vi "ForceGraph(Position).vi"(8 "number":dbl, 9 "Setpoint":dbl, 10 "k":dbl, 11 "Function":string) -> (1 "force":dbl)   [LabVIEW 2023]
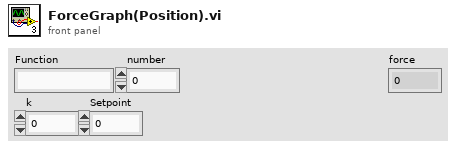
[diagram p1: front panel]
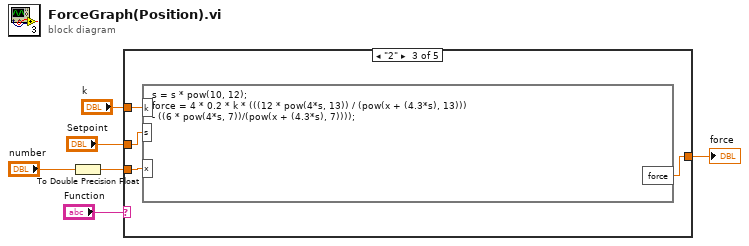
[diagram p0: block diagram]
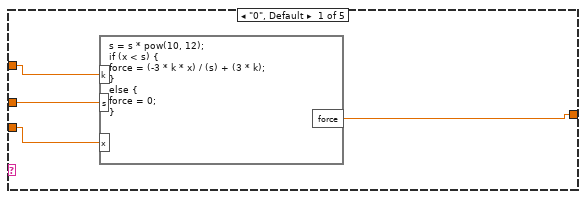
[diagram p2: hidden frame]
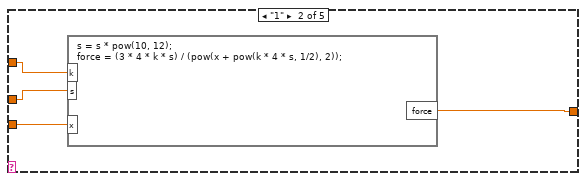
[diagram p3: hidden frame]
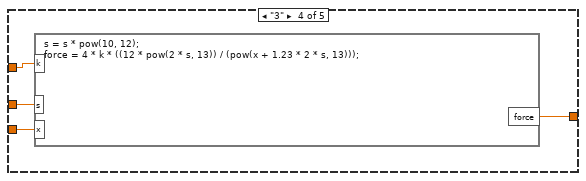
[diagram p4: hidden frame]
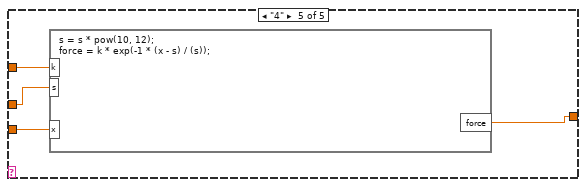
[diagram p5: hidden frame]
diagram:
  n1 = To Double Precision Float(number="number") -> (double precision float=w3:dbl)
  n2 = case shown="\"2\"" "Function" {
    tunnel: [w9 w13 w17 w22 w25] -> w1
    tunnel: w3 -> [w10 w14 w18 w21 w26]
    tunnel: "Setpoint" -> [w8 w11 w15 w19 w23]
    tunnel: "k" -> [w7 w12 w16 w20 w24]
    frame "0", Default {
      n3 = formula code="s = s * pow(10, 12);\nif (x < s) {\nforce = (-3 * k * x) / (s) + (3 * k);\n}\nelse {\nforce = 0;\n}"("k"=w7, "s"=w8, "x"=w10) -> ("force"=w9:dbl)
    }
    frame "1" {
      n4 = formula code="s = s * pow(10, 12);\nforce = (3 * 4 * k * s) / (pow(x + pow(k * 4 * s, 1/2), 2));"("k"=w12, "s"=w11, "x"=w14) -> ("force"=w13:dbl)
    }
    frame "2" {
      n5 = formula code="s = s * pow(10, 12);\nforce = 4 * 0.2 * k * (((12 * pow(4*s, 13)) / (pow(x + (4.3*s), 13))) \n- ((6 * pow(4*s, 7))/(pow(x + (4.3*s), 7))));"("x"=w18, "s"=w15, "k"=w16) -> ("force"=w17:dbl)
    }
    frame "3" {
      n6 = formula code="s = s * pow(10, 12);\nforce = 4 * k * ((12 * pow(2 * s, 13)) / (pow(x + 1.23 * 2 * s, 13)));"("k"=w20, "s"=w19, "x"=w21) -> ("force"=w22:dbl)
    }
    frame "4" {
      n7 = formula code="s = s * pow(10, 12);\nforce = k * exp(-1 * (x - s) / (s));"("k"=w24, "s"=w23, "x"=w26) -> ("force"=w25:dbl)
    }
  }
  "force" <- w1
